vi "Condition Type.vi"(11 "Expression Condition Config in":refnum<class "Expression Condition Config.lvclass">) -> (2 "Condition Type":string)   [LabVIEW 2020, in "VolatusSeqConfig.lvlib" / "Expression Condition Config.lvclass"]
uses:
  Expression Condition Config.lvclass
  Expression Condition Config.lvclass/Expression Condition Config.ctl
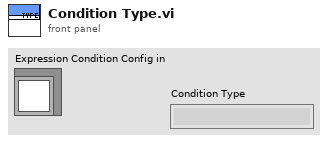
[diagram p1: front panel]
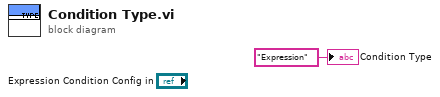
[diagram p0: block diagram]
diagram:
  "Condition Type" <- "Expression" ("Condition Type")
